vi "SCT Update Controls.vi"(0 "Variable Dialog Controls":T1, 1 "SCT Update Controls Flags":T2, 2 "Project Refnum":refnum<vi>, 5 "Dialog Edit State in":T14, 7 "Variables in":T3[](array[typedef]), 9 "state variables in":T6, 11 "error in (no error)":errorcluster, 12 "feature pack info":T10, 13 "default types":T13, 14 "Items To Apply":i32[](array[numeric])) -> (3 "valid?":bool, 4 "Variable Dialog Controls out":T1, 6 "Dialog Edit State out":T14, 8 "Variables out":T3[](array[typedef]), 10 "state variables out":T6, 15 "error out":errorcluster)   [LabVIEW 2016]
uses:
  <resource>/dialog/variable/SCT Variable.ctl
  <vilib>/variable/Type Descriptor.ctl
  <vilib>/variable/Attribs.ctl
  <resource>/dialog/variable/SCT Dialog Single Source Edit State.ctl
  <resource>/dialog/variable/SCT Default Types.ctl
  <resource>/dialog/variable/SCT State Variables.ctl
  <resource>/dialog/variable/SCT Feature State.ctl
  <resource>/dialog/variable/SCT Variable Changes.ctl
  <resource>/dialog/variable/SCT Attribute Changes.ctl
  <resource>/dialog/variable/SCT Feature Pack Info.ctl
  <resource>/dialog/variable/SCT Message User Event.ctl
  <resource>/dialog/variable/SCT Message.ctl
  <resource>/dialog/variable/SCT Attributes.ctl
  <resource>/dialog/variable/SCT Attributes Event.ctl
  <resource>/dialog/variable/SCT Variable Dialog Controls.ctl
  <resource>/dialog/variable/SCT Update Controls Flags.ctl
  <vilib>/variable/NI_Variable.lvlib
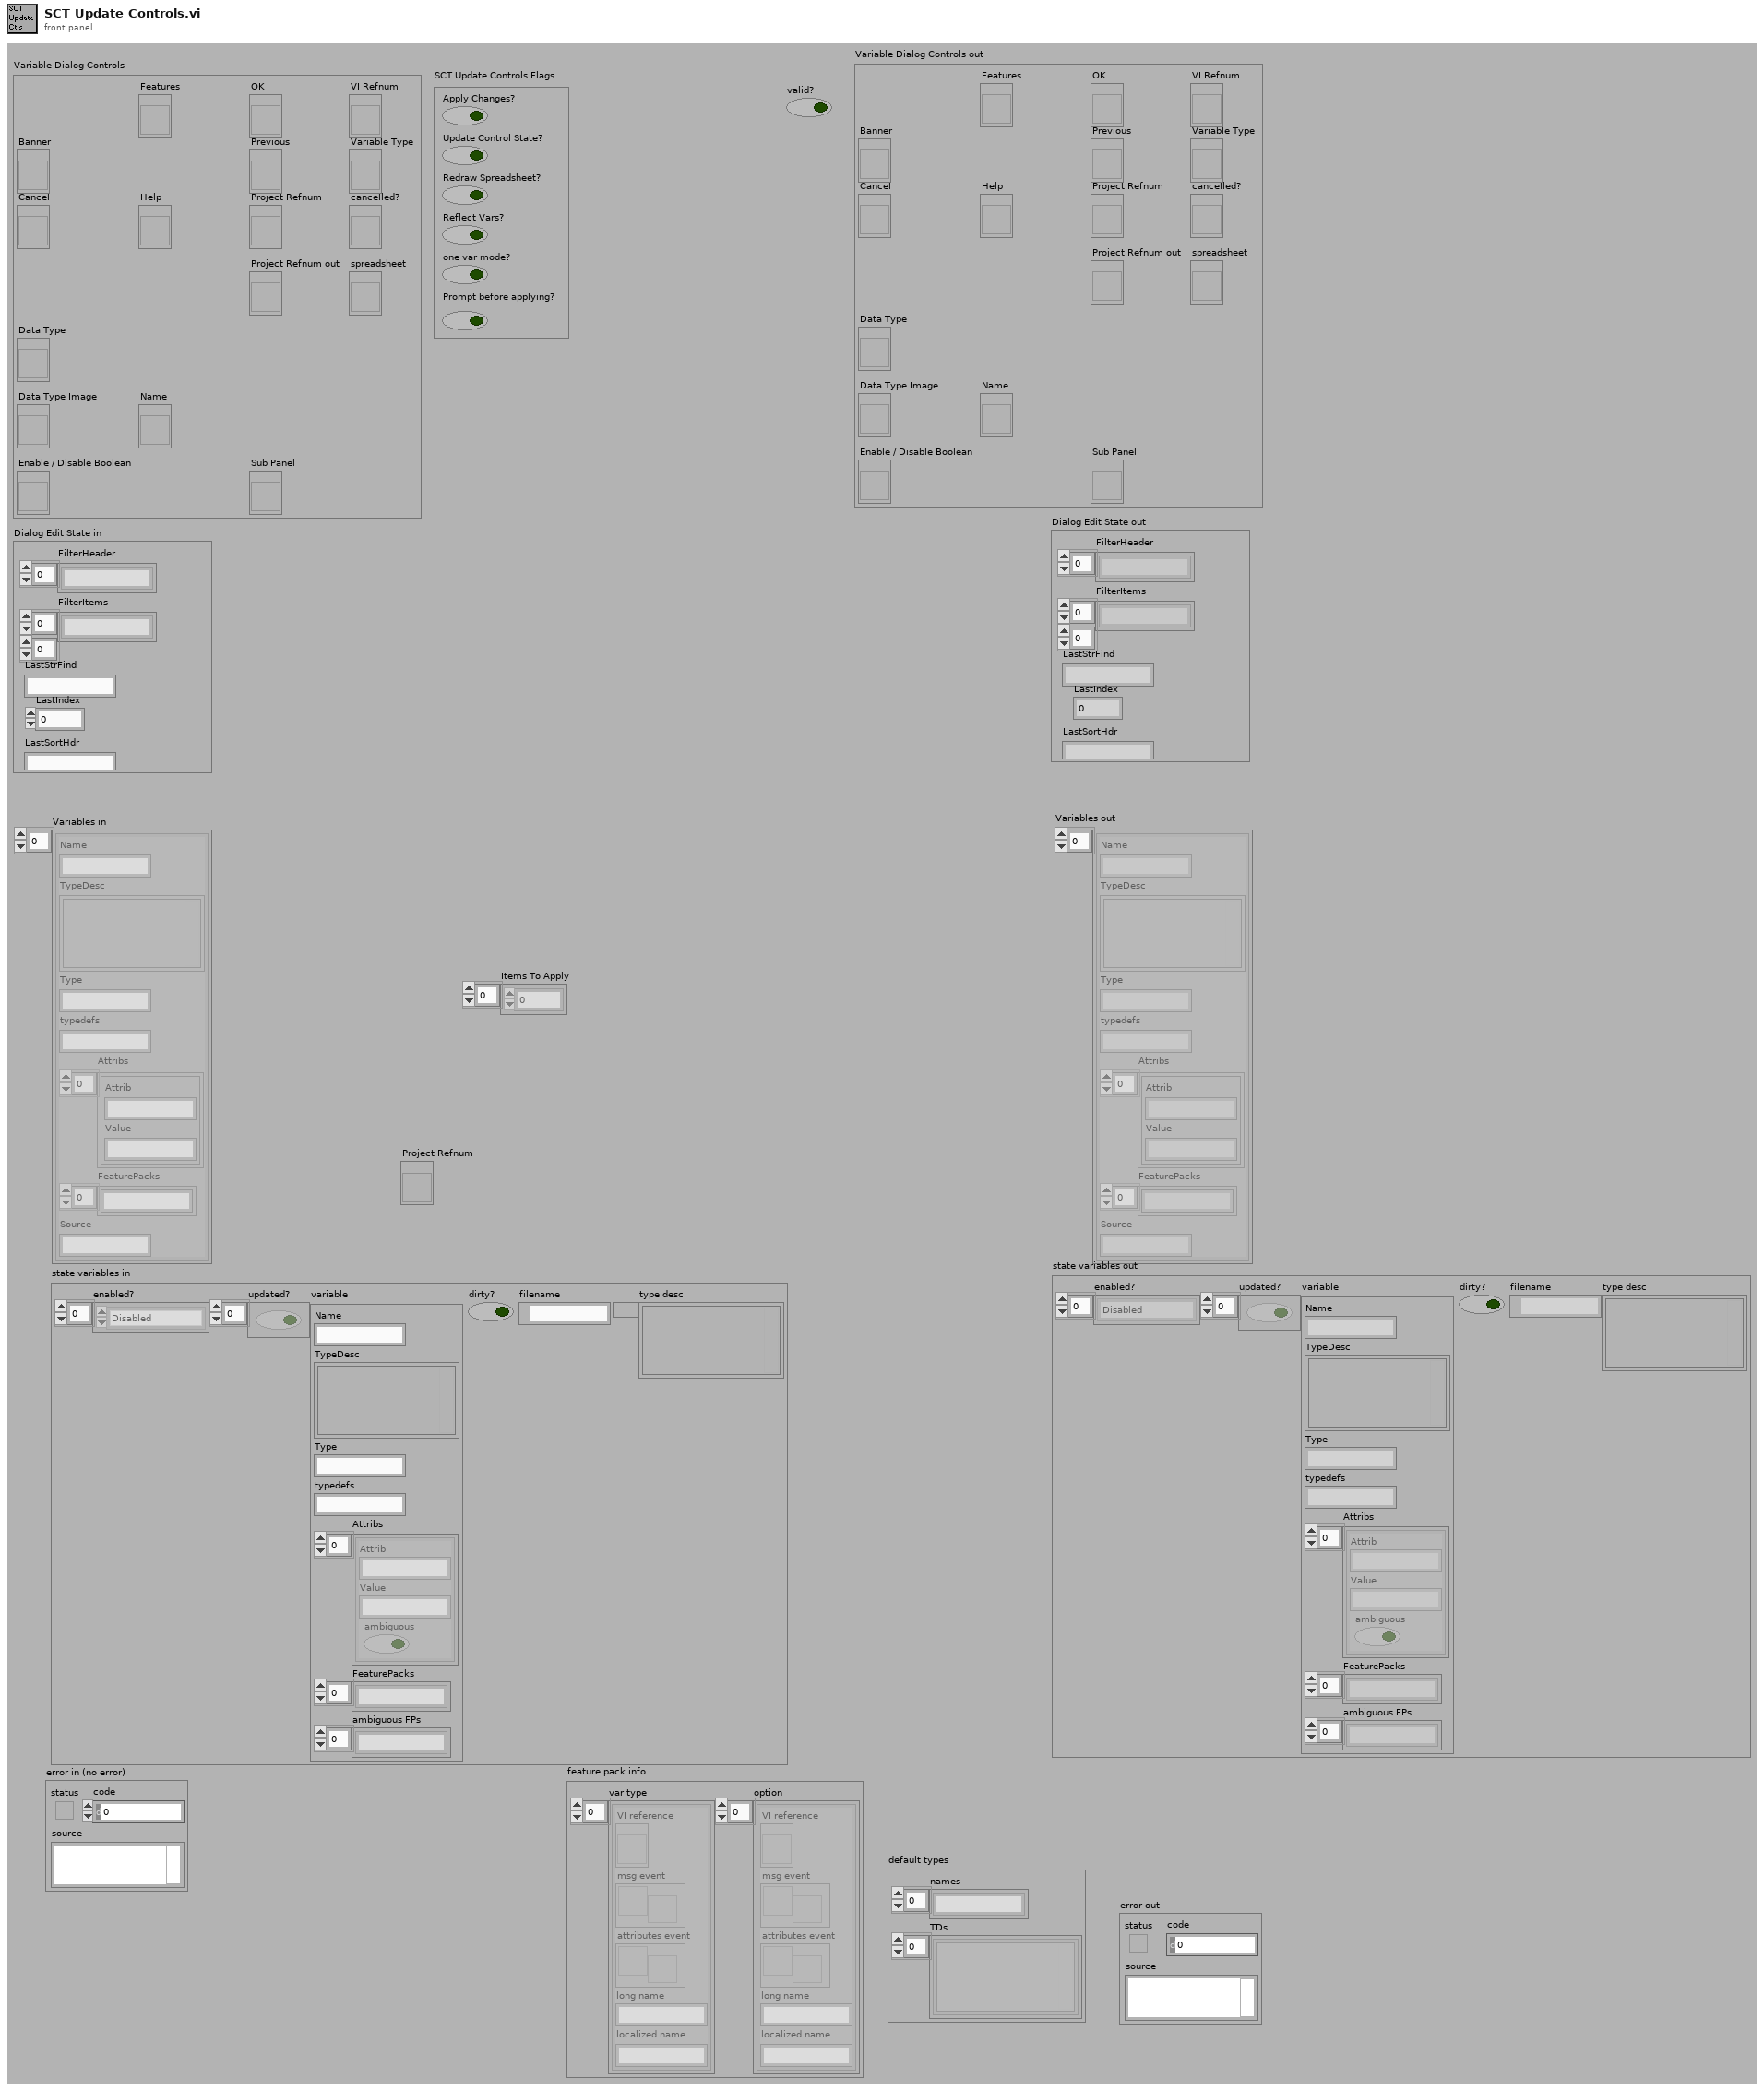
[diagram p1: front panel]
types:
  T1 = typedef "SCT Variable Dialog Controls.ctl" = cluster{"Banner":refnum<vi>, "Cancel":refnum<vi>, "Data Type":refnum<vi>, "Data Type Image":refnum<vi>, "Enable / Disable Boolean":refnum<vi>, "Features":refnum<vi>, "Help":refnum<vi>, "Name":refnum<vi>, "OK":refnum<vi>, "Previous":refnum<vi>, "Project Refnum":refnum<vi>, "Project Refnum out":refnum<vi>, "Sub Panel":refnum<vi>, "VI Refnum":refnum<vi>, "Variable Type":refnum<vi>, "cancelled?":refnum<vi>, "spreadsheet":refnum<vi>}
  T2 = typedef "SCT Update Controls Flags.ctl" = cluster{"Apply Changes?":bool, "Update Control State?":bool, "Redraw Spreadsheet?":bool, "Reflect Vars?":bool, "one var mode?":bool, "Prompt before applying?":bool}
  T3 = typedef "SCT Variable.ctl" = cluster{"Name":string, "TypeDesc":T4, "Type":string, "typedefs":string, "Attribs":T5, "FeaturePacks":string[], "Source":string}
  T4 = typedef "NI_Variable.lvlib/Type Descriptor.ctl" = cluster{"Variant":variant}
  T5 = typedef "NI_Variable.lvlib/Attribs.ctl" = cluster{"Attrib":string, "Value":string}[]
  T6 = typedef "SCT State Variables.ctl" = cluster{"enabled?":T7[], "updated?":bool[], "variable":T8, "dirty?":bool, "filename":path, "type desc":T4}
  T7 = typedef "SCT Feature State.ctl" = enum16{"Disabled", "Enabled", "Ambiguous", "Grayed", "MultiSelectConst"}
  T8 = typedef "SCT Variable Changes.ctl" = cluster{"Name":string, "TypeDesc":T4, "Type":string, "typedefs":string, "Attribs":T9, "FeaturePacks":string[], "ambiguous FPs":string[]}
  T9 = typedef "SCT Attribute Changes.ctl" = cluster{"Attrib":string, "Value":string, "ambiguous":bool}[]
  T10 = typedef "SCT Feature Pack Info.ctl" = cluster{"var type":cluster{"VI reference":refnum<vi>, "msg event":T11, "attributes event":T12, "long name":string, "localized name":string}[], "option":cluster{"VI reference":refnum<vi>, "msg event":T11, "attributes event":T12, "long name":string, "localized name":string}[]}
  T11 = typedef "SCT Message User Event.ctl" = refnum<user-event>
  T12 = typedef "SCT Attributes Event.ctl" = refnum<user-event>
  T13 = typedef "SCT Default Types.ctl" = cluster{"names":string[], "TDs":T4[]}
  T14 = typedef "SCT Dialog Single Source Edit State.ctl" = cluster{"FilterHeader":string[], "FilterItems":string[][], "LastStrFind":string, "LastIndex":i32, "LastSortHdr":string}
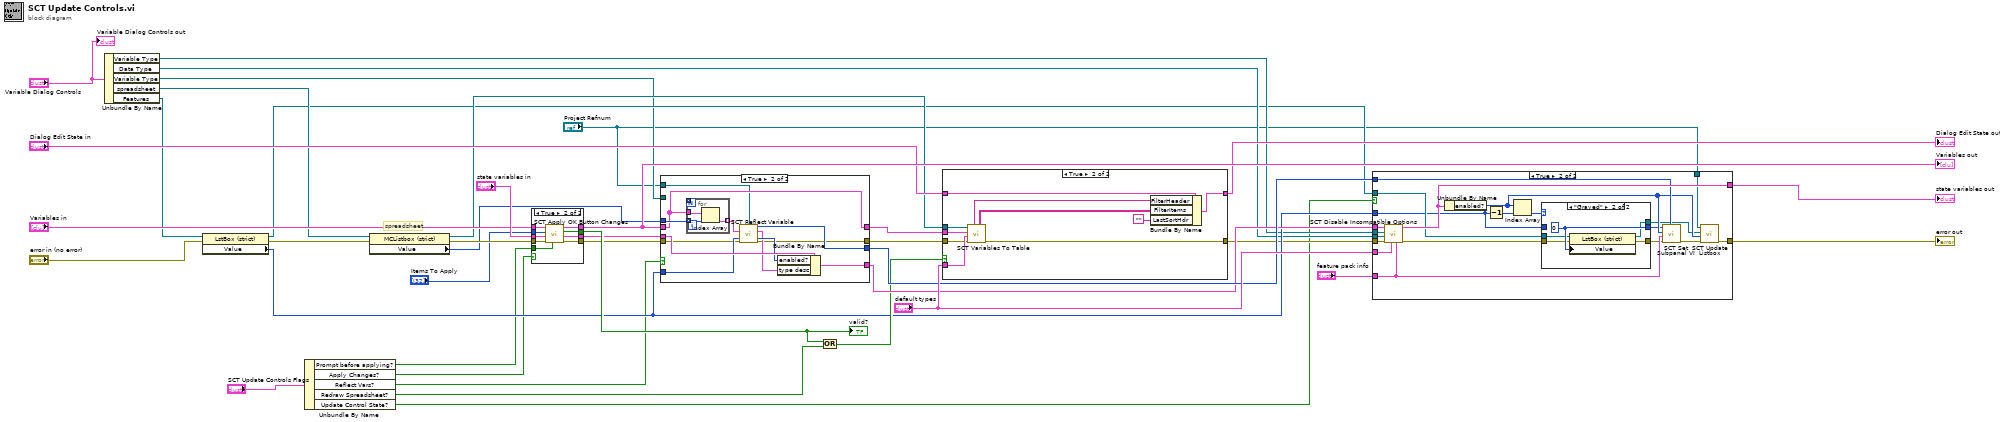
[diagram p0: block diagram]
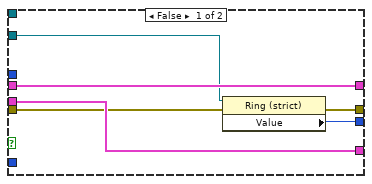
[diagram p4: hidden frame]
diagram:
  # "spreadsheet"
  n1 = Unbundle By Name("Variable Dialog Controls") -> ("Variable Type"=w17:refnum<vi>, "Data Type"=w24:refnum<vi>, "Variable Type"=w12:refnum<vi>, "spreadsheet"=w16:refnum<vi>, "Features"=w14:refnum<vi>)
  n2 = property class="LstBox (strict)"(reference=w14, error in="error in (no error)") -> (reference out=w13:refnum<vi>, error out=w15:errorcluster, "Value"=w25:i32)
  n3 = Unbundle By Name("SCT Update Controls Flags") -> ("Prompt before applying?"=w4:bool, "Apply Changes?"=w10:bool, "Reflect Vars?"=w9:bool, "Redraw Spreadsheet?"=w8:bool, "Update Control State?"=w7:bool)
  n4 = property class="MCListbox (strict)"(reference=w16, error in=w15) -> (reference out=w23:refnum<vi>, error out=w22:errorcluster, "Value"=w3:i32[])
  n5 = case shown="True" w10 {
    selector: w10 -> [w43 _]
    tunnel: [w43 w48] -> w37
    tunnel: "Variables in" -> [w42 w52]
    tunnel: [w42 w51] -> w38
    tunnel: "state variables in" -> [w41 w49]
    tunnel: [w41 w50] -> w28
    tunnel: "Items To Apply" -> [_ w45]
    tunnel: w22 -> [w40 w47]
    tunnel: [w40 w46] -> w21
    tunnel: w4 -> [_ w44]
    frame False {
    }
    frame True {
      n6 = call <resource>:"SCT Apply OK Button Changes.vi"("Prompt?"=w44, "error in (no error)"=w47, "state variables in"=w49, "spreadsheet lines selected"=w45, "variables"=w52) -> ("error out"=w46:errorcluster, "state variables out"=w50:T6, "valid?"=w48:bool, "updated vars"=w51:T3[])  [unwired: 3 in]
    }
  }
  "Variables out" <- w38
  "valid?" <- w37
  n7 = case shown="True" w9 {
    tunnel: w28 -> [w58 w70]
    tunnel: [w58 w69] -> w31
    tunnel: w38 -> [w56 w63]
    tunnel: w3 -> [_ w68]
    tunnel: [w57 w64] -> w33
    tunnel: [w56 w63] -> w39
    tunnel: w25 -> [_ w62]
    tunnel: w21 -> [w55 w60]
    tunnel: [w54 w61] -> w20
    tunnel: w12 -> [w53 _]
    tunnel: "Project Refnum" -> [_ w59]
    frame False {
      n8 = property class="Ring (strict)"(reference=w53, error in=w55) -> (error out=w54:errorcluster, "Value"=w57:i32)  [unwired: 1 out]
    }
    frame True {
      n9 = for {
        N -> [w71]
        tunnel: w63 -> [w74]
        tunnel: w68 -> [w73] mode=indexing
        tunnel: [w72] -> w67 mode=indexing
        tunnel: [w71] -> _ mode=indexing
        n10 = Index Array(array=w74, index=w73) -> (element=w72:T3)
      }
      n11 = call <resource>:"SCT Reflect Variable.vi"("Project Refnum"=w59, "variables to reflect"=w67, "listbox index"=w62, "error in (no error)"=w60) -> ("var type index"=w64:i32, "type descriptor"=w65:T4, "options enabled"=w66:enum16{"Disabled", "Enabled", "Ambiguous"}[], "error out"=w61:errorcluster)  [unwired: 8 in]
      n12 = Bundle By Name(cluster=w70, "enabled?"=w66, "type desc"=w65) -> (w69:T6)
    }
  }
  n13 = Or(x=w37, y=w8) -> (x .or. y?=w27:bool)
  n14 = case shown="True" w27 {
    tunnel: w39 -> [_ w86]
    tunnel: "default types" -> [_ w85]
    tunnel: "Dialog Edit State in" -> [w76 w84]
    tunnel: [w76 w83] -> w36
    tunnel: w23 -> [_ w79]
    tunnel: w20 -> [w75 w78]
    tunnel: [w75 w77] -> w19
    frame False {
    }
    frame True {
      n15 = call <resource>:"SCT Variables To Table.vi"("error in (no error)"=w78, "default types"=w85, "variables"=w86, "spreadsheet"=w79) -> ("error out"=w77:errorcluster, "Filtered Table"=w81:string[][], "Filtered Header"=w82:string[])  [unwired: 3 in, 2 out]
      n16 = Bundle By Name(cluster=w84, "FilterHeader"=w82, "FilterItems"=w81, "LastSortHdr"="") -> (w83:T14)
    }
  }
  "Dialog Edit State out" <- w36
  n17 = case shown="True" w7 {
    tunnel: [w88 w106] -> w18
    tunnel: w31 -> [w88 w108]
    tunnel: "default types" -> [_ w107]
    tunnel: "feature pack info" -> [_ w93]
    tunnel: w33 -> [_ w105]
    tunnel: w13 -> [_ w99]
    tunnel: w25 -> [_ w98]
    tunnel: w17 -> [_ w96]
    tunnel: w24 -> [_ w95]
    tunnel: w19 -> [w87 w94]
    tunnel: [w87 w90] -> w6
    tunnel: "Project Refnum" -> [_ w89]
    frame False {
    }
    frame True {
      n18 = call <resource>:"SCT Disable Incompatible Options.vi"("feature pack info"=w93, "default types"=w107, "error in (no error)"=w94, "data type"=w95, "variable type"=w96, "state variables"=w108) -> ("error out"=w92:errorcluster, "state variables out"=w106:T6)  [unwired: 4 in]
      n19 = Unbundle By Name(w106) -> ("enabled?"=w103:T7[])
      n20 = Decrement(x=w98) -> (x-1=w102:i32)
      n21 = Index Array(array=w103, index=w102) -> (element=w101:T7)
      n22 = case shown="\"Grayed\"" w101 {
        tunnel: [w111 w116] -> w100
        tunnel: w98 -> [w111 _]
        tunnel: w99 -> [w110 w115]
        tunnel: [w110 w114] -> w97
        tunnel: w92 -> [w109 w113]
        tunnel: [w109 w112] -> w91
        frame Default {
        }
        frame "Grayed" {
          w116 = 0
          n23 = property class="LstBox (strict)"(reference=w115, error in=w113, "Value"=w116) -> (reference out=w114:refnum<vi>, error out=w112:errorcluster)
        }
      }
      n24 = call <resource>:"SCT Set Subpanel VI.vi"("var type index"=w105, "error in (no error)"=w91, "feature pack info"=w93, "enabled array"=w103, "listbox index"=w100) -> ("error out"=w104:errorcluster)  [unwired: 6 in]
      n25 = call <resource>:"SCT Update Listbox.vi"("error in (no error)"=w104, "enabled"=w103, "feature listbox"=w97, "Project Refnum"=w89) -> ("error out"=w90:errorcluster)  [unwired: 7 in]
    }
  }
  "state variables out" <- w18
  "error out" <- w6
  "Variable Dialog Controls out" <- "Variable Dialog Controls"
